vi "Handle Command.vi"(8 "error in":errorcluster, 10 "Change TEC Enables in":refnum<class "Change TEC Enables.lvclass">, 11 "Object In":refnum<class>) -> (0 "error out":errorcluster, 1 "Command Successful?":bool, 2 "Change TEC Enables out":refnum<class "Change TEC Enables.lvclass">, 3 "Object Out":refnum<class>)   [LabVIEW 2014, in "Change TEC Enables.lvclass"]
doc: "Abstract method for accomplishing the execution of a command directed to an instrument object on the wire."
uses:
  Change TEC Enables.lvclass
  Instrument/ePAS.lvclass
  reusable/Session APIs/Session Log/System Log.lvclass
  <vilib>/DAQmx/write.llb/DAQmx Write (Digital 1D Bool NChan 1Samp 1Line).vi
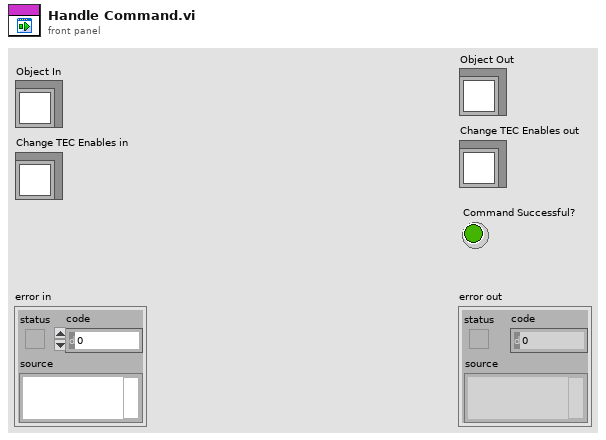
[diagram p1: front panel]
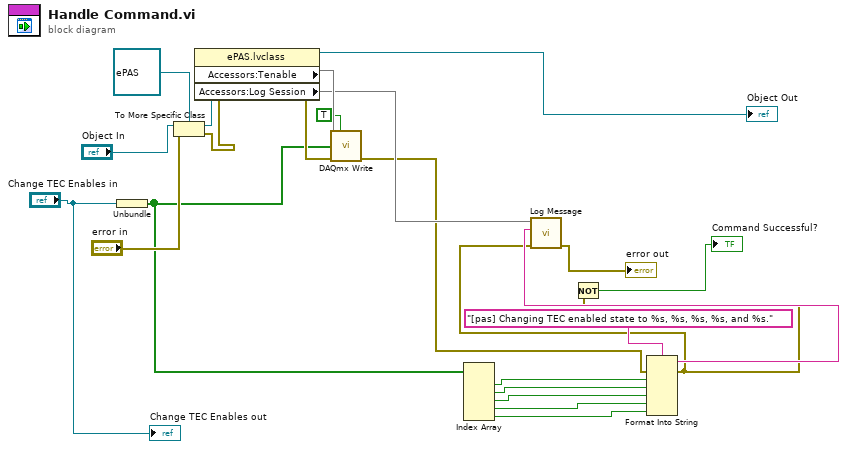
[diagram p0: block diagram]
diagram:
  n1 = Unbundle("Change TEC Enables in") -> (w4:bool[])
  n2 = To More Specific Class(target class=refnum<class "ePAS.lvclass"> refnum ("ePAS"), reference="Object In", error in="error in") -> (specific class reference=w20:refnum<class "ePAS.lvclass">, error out=w19:errorcluster)
  n3 = property class="ePAS.lvclass"(reference=w20, error in=w19) -> (reference out=→"Object Out":refnum<class "ePAS.lvclass">, error out=w18:errorcluster, "Accessors:Tenable"=w17, "Accessors:Log Session"=w16)
  n4 = call-poly <vilib>:"DAQmx Write.vi"("task/channels in"=w17, "auto start"=TRUE, "data"=w4, "error in"=w18) -> ("error out"=w8:errorcluster)  [unwired: 9 in, 2 out]
  n5 = Index Array(array=w4) -> (element #1=w14:bool, element #2=w13:bool, element #3=w12:bool, element #4=w11:bool, element #5=w10:bool)  [unwired: 5 in]
  n6 = Format Into String(format string="[pas] Changing TEC enabled state to %s, %s, %s, %s, and %s.", error in=w8, w14, w13, w12, w11, w10) -> (resulting string=w9:string, error out=w2:errorcluster)  [unwired: 1 in]
  n7 = call "Log Message.vi"("error in"=w2, "MSG In"=w9, "session in"=w16) -> ("error out"=→"error out":errorcluster)  [unwired: 7 in, 1 out]
  n8 = Not(x=w2) -> (.not. x?=→"Command Successful?":bool)
  "Change TEC Enables out" <- "Change TEC Enables in"
